vi "Resistance Measurements.vi"() -> ()   [LabVIEW 2017]
uses:
  <instrlib>/Keithley 24XX/Public/Data/Read (Multiple Points).vi
  <vilib>/Utility/file.llb/Write Delimited Spreadsheet (string).vi
  <instrlib>/Keithley 24XX/Keithley 24XX.lvlib
  <vilib>/Analysis/NI_AALPro.lvlib
panel:
  out "Boolean":bool
  out "Current Sample":dbl
  out "Beam State":bool
  in  "Beam Switch":bool
  in  "Samples per toggle":dbl=6.0
  in  "Toggle Beam":bool
  in  "File Suffix":string
  in  "File Prefix":string
  in  "File Directory":path
  out "IV Curve":cluster{"Y":dbl[], "Y":dbl[]}[](graph)
  in  "Stopped":bool
  in  "Milliseconds per sample":u32=180000
  in  "Source Mode  (0: Voltage)":u16(ring) items=["Voltage", "Current"]
  in  "Serial Configuration":T1={"Baud Rate"=9600, "Parity"=0, "Data Bits"=8, "Stop Bits"=10, "Flow Control"=0} {"Flow Control" items=["None", "XON/XOFF", "RTS/CTS", "XON/XOFF & RTS/CTS", "DTR/DSR", "XON/XOFF & DTR/DSR"]; "Stop Bits" items=["1.0"=10, "1.5"=15, "2.0"=20]; "Data Bits" items=["7"=7, "8"=8]; "Parity" items=["None", "Odd", "Even", "Mark", "Space"]; "Baud Rate" items=["300"=300, "600"=600, "1200"=1200, "2400"=2400, "4800"=4800, "9600"=9600, "19200"=19200]}
  in  "VISA resource name":refnum<visa-resource-name>
  in  "Timeout (10000 ms)":i32=30000 format="%#.6g"
  in  "Maximum Amplitude (2)":dbl=0.1
  in  "Minimum Amplitude (1)":dbl=-0.1
  in  "Number of Points (5)":u32=20
  in  "Compliance  Level (0.1)":dbl=0.1
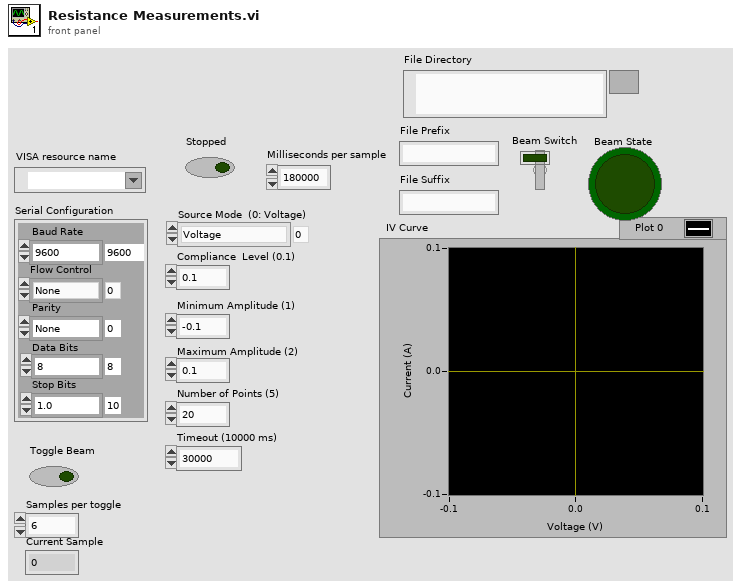
[diagram p1: front panel]
types:
  T1 = cluster{"Baud Rate":u32, "Parity":u16, "Data Bits":u16, "Stop Bits":u16, "Flow Control":u16}
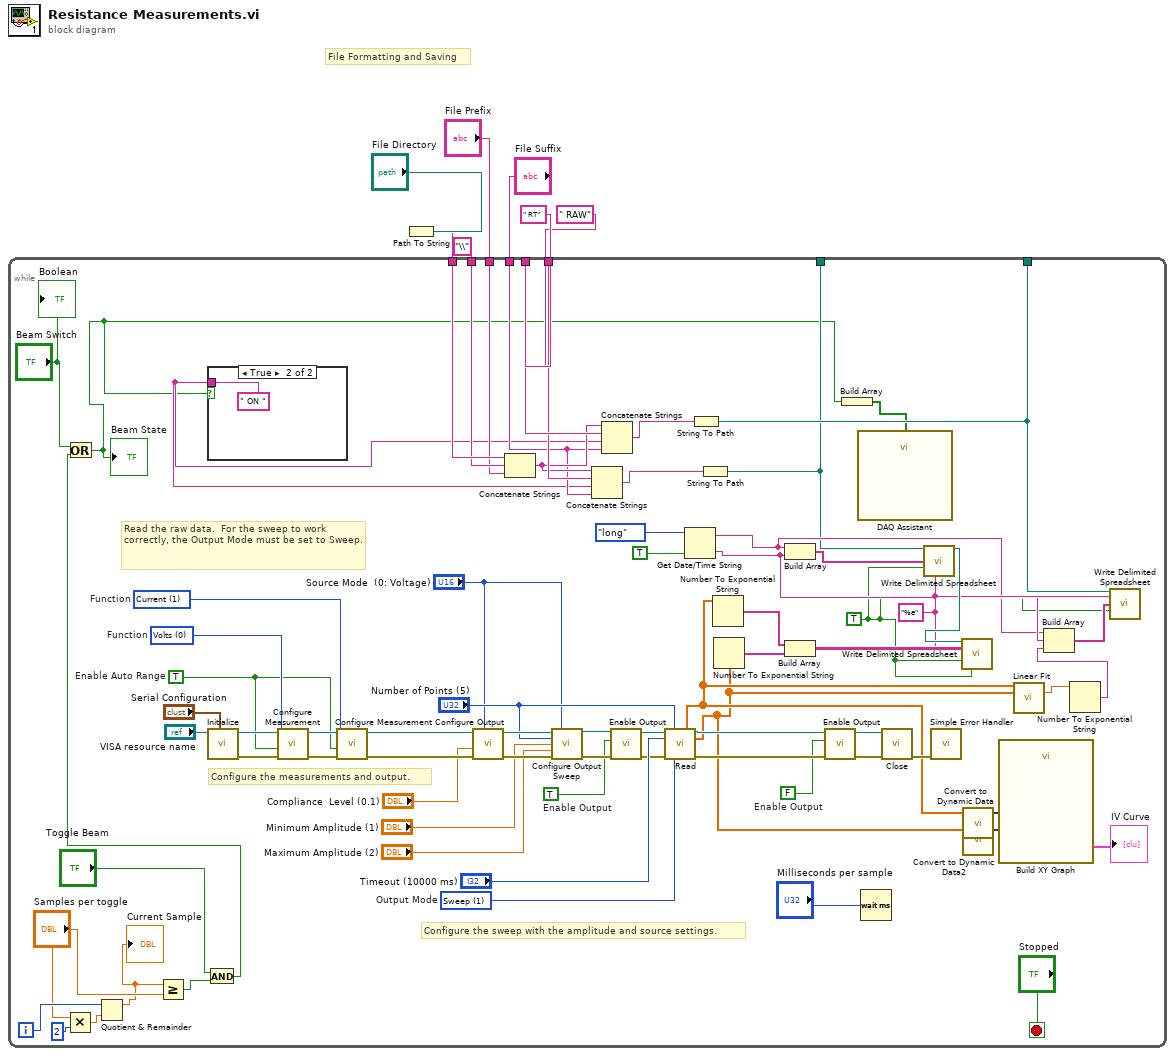
[diagram p0: block diagram]
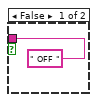
[diagram p2: hidden frame]
diagram:
  # "File Formatting and Saving"
  n1 = Path To String(path="File Directory") -> (string=w6:string)
  n2 = while {
    tunnel: [w20] -> _
    tunnel: [w22] -> _
    tunnel: w6 -> [w30]
    tunnel: "File Prefix" -> [w28]
    tunnel: "\\" -> [w29]
    tunnel: "File Suffix" -> [w24]
    tunnel: " RT" -> [w27]
    tunnel: " RAW" -> [w26]
    i -> [w17]
    stop <- "Stopped" stop-if-true
    w37 = TRUE
    w43 = "%e"
    w53 = TRUE  # Enable Output
    w54 = TRUE  # Enable Auto Range
    w55 = u16 1 items=["Volts", "Current", "Resistance"]  # Function
    w56 = u16 0 items=["Volts", "Current", "Resistance"]  # Function
    w62 = FALSE  # Enable Output
    w68 = u16 1 items=["Fixed", "Sweep", "List"]  # Output Mode
    # "Read the raw data.  For the sweep to work correctly, the Output Mode must be set to Sweep."
    # "Configure the sweep with the amplitude and source settings."
    # "Configure the measurements and output."
    n3 = Multiply(x="Samples per toggle", y=2) -> (x*y=w14:dbl)
    n4 = Quotient & Remainder(x=w17, y=w14) -> (x-y*floor(x/y)=w11:dbl)  [unwired: 1 out]
    "Current Sample" <- w11
    n5 = Greater Or Equal?(x=w11, y="Samples per toggle") -> (x >= y?=w12:bool)
    n6 = And(x="Toggle Beam", y=w12) -> (x .and. y?=w10:bool)
    n7 = Or(x="Beam Switch", y=w10) -> (x .or. y?=w9:bool)
    "Beam State" <- w9
    n8 = case shown="True" w9 {
      tunnel: [" OFF " " ON "] -> w18
      frame False {
      }
      frame True {
      }
    }
    n9 = call <instrlib>:"Initialize.vi"("Serial Configuration"="Serial Configuration", "VISA resource name"="VISA resource name") -> ("error out"=w81:errorcluster, "VISA resource name out"=w82:refnum<visa-resource-name>)  [unwired: 8 in]
    n10 = call <instrlib>:"Configure Measurement.vi"("error in (no error)"=w81, "Enable Auto Range (T:Enable)"=w54, "Function (0: Volts)"=w56, "VISA resource name"=w82) -> ("error out"=w80:errorcluster, "VISA resource name out"=w79:refnum<visa-resource-name>)  [unwired: 6 in]
    n11 = call <instrlib>:"Configure Measurement.vi"("error in (no error)"=w80, "Enable Auto Range (T:Enable)"=w54, "Function (0: Volts)"=w55, "VISA resource name"=w79) -> ("error out"=w77:errorcluster, "VISA resource name out"=w78:refnum<visa-resource-name>)  [unwired: 6 in]
    n12 = call <instrlib>:"Configure Output.vi"("Source Mode  (0: Voltage)"="Source Mode  (0: Voltage)", "error in (no error)"=w77, "Compliance  Level (0.1)"="Compliance  Level (0.1)", "VISA resource name"=w78) -> ("error out"=w76:errorcluster, "VISA resource name out"=w75:refnum<visa-resource-name>)  [unwired: 6 in]
    n13 = Concatenate Strings(w30, w29, w28) -> (w25:string)
    n14 = call <instrlib>:"Configure Output Sweep.vi"("VISA resource name"=w75, "Source Mode  (0: Voltage)"="Source Mode  (0: Voltage)", "Number of Points (5)"="Number of Points (5)", "Minimum Amplitude (1)"="Minimum Amplitude (1)", "Maximum Amplitude (2)"="Maximum Amplitude (2)", "error in (no error)"=w76) -> ("VISA resource name out"=w59:refnum<visa-resource-name>, "error out"=w58:errorcluster)  [unwired: 8 in]
    n15 = Concatenate Strings(w25, w26, w18, w24) -> (w21:string)
    n16 = Concatenate Strings(w25, w27, w18, w24) -> (w23:string)
    n17 = call <instrlib>:"Enable Output.vi"("error in (no error)"=w58, "Enable Output (T: Enable)"=w53, "VISA resource name"=w59) -> ("error out"=w61:errorcluster, "VISA resource name out"=w60:refnum<visa-resource-name>)  [unwired: 7 in]
    n18 = call-poly <instrlib>:"Read.vi"("VISA resource name"=w60, "Sample Count (1)"="Number of Points (5)", "Timeout (10000 ms)"="Timeout (10000 ms)", "error in (no error)"=w61, "Output Mode (0: Fixed)"=w68) -> ("Voltage"=w34:sgl[], "VISA resource name out"=w63:refnum<visa-resource-name>, "Current"=w32:sgl[], "error out"=w64:errorcluster)  [unwired: 4 in, 3 out]
    n19 = Get Date/Time String(date format (0)=enum16{"short", "long", "abbreviated"}."long", want seconds? (F)=TRUE) -> (date string=w40:string, time string=w41:string)  [unwired: 1 in]
    n20 = String To Path(string=w23) -> (path=w22:path)
    n21 = String To Path(string=w21) -> (path=w20:path)
    n22 = Number To Exponential String(number=w34) -> (E-format string=w47:string[])  [unwired: 3 in]
    n23 = Number To Exponential String(number=w32) -> (E-format string=w48:string[])  [unwired: 3 in]
    n24 = Build Array(w40, w41) -> (w46:string[])
    n25 = Build Array(w47, w48) -> (w45:string[][])
    n26 = call <instrlib>:"Enable Output.vi"("error in (no error)"=w64, "Enable Output (T: Enable)"=w62, "VISA resource name"=w63) -> ("error out"=w65:errorcluster, "VISA resource name out"=w66:refnum<visa-resource-name>)  [unwired: 7 in]
    n27 = Build Array(w9) -> (w19:bool[])
    n28 = call "DAQ Assistant"("data"=w19) -> ()  [unwired: 17 in, 2 out]
    n29 = Wait (ms)(milliseconds to wait="Milliseconds per sample") -> ()  [unwired: 1 out]
    n30 = call <instrlib>:"Close.vi"("error in (no error)"=w65, "VISA resource name"=w66) -> ("error out"=w67:errorcluster)  [unwired: 9 in]
    n31 = call-poly <vilib>:"Write Delimited Spreadsheet.vi"("file path (dialog if empty)"=w20, "format (%s)"=w43, "1D data"=w46, "append to file? (new file:F)"=w37) -> ("new file path (Not A Path if cancelled)"=w44:path)  [unwired: 10 in, 1 out]
    n32 = call <vilib>:"Simple Error Handler.vi"("error in (no error)"=w67) -> ()  [unwired: 4 in, 5 out]
    n33 = call-poly <vilib>:"Write Delimited Spreadsheet.vi"("file path (dialog if empty)"=w44, "format (%s)"=w43, "2D data"=w45, "append to file? (new file:F)"=w37, "transpose? (no:F)"=w37) -> ()  [unwired: 9 in, 2 out]
    n34 = call "Convert to Dynamic Data"("Array"=w34) -> ("Dynamic Data Type"=w33:dynamicdata)  [unwired: 3 in]
    n35 = call "Convert to Dynamic Data2"("Array"=w32) -> ("Dynamic Data Type"=w31:dynamicdata)  [unwired: 3 in]
    n36 = call "Build XY Graph"("Y Input"=w31, "X Input"=w33) -> ("XY Graph"=→"IV Curve":cluster{"X":dbl[], "Y":dbl[]}[])  [unwired: 8 in, 1 out]
    n37 = call <vilib>:"Linear Fit.vi"("Y"=w34, "X"=w32) -> ("slope"=w42:dbl)  [unwired: 9 in, 4 out]
    n38 = Number To Exponential String(number=w42) -> (E-format string=w39:string)  [unwired: 3 in]
    n39 = Build Array(w40, w41, w39) -> (w38:string[])
    n40 = call-poly <vilib>:"Write Delimited Spreadsheet.vi"("file path (dialog if empty)"=w22, "format (%s)"=w43, "1D data"=w38, "append to file? (new file:F)"=w37) -> ()  [unwired: 10 in, 2 out]
    "Boolean" <- "Beam Switch"
  }
